vi "stopSel.vi"(5 "Der Ampl":dbl, 6 "Tipo":enum16{"Amplitud", "Fase", "Mixto"}(ring), 7 "Der Fase":dbl, 8 "thr":dbl, 9 "thr. Ang":dbl, 10 "Err.Amp":dbl, 11 "DifFase":dbl) -> (2 "stop":bool)   [LabVIEW 2018]
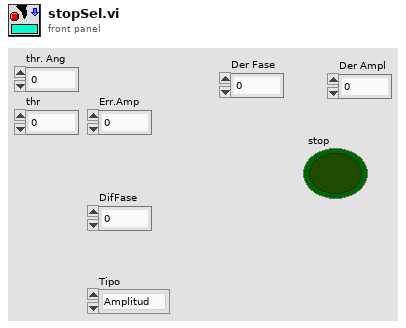
[diagram p1: front panel]
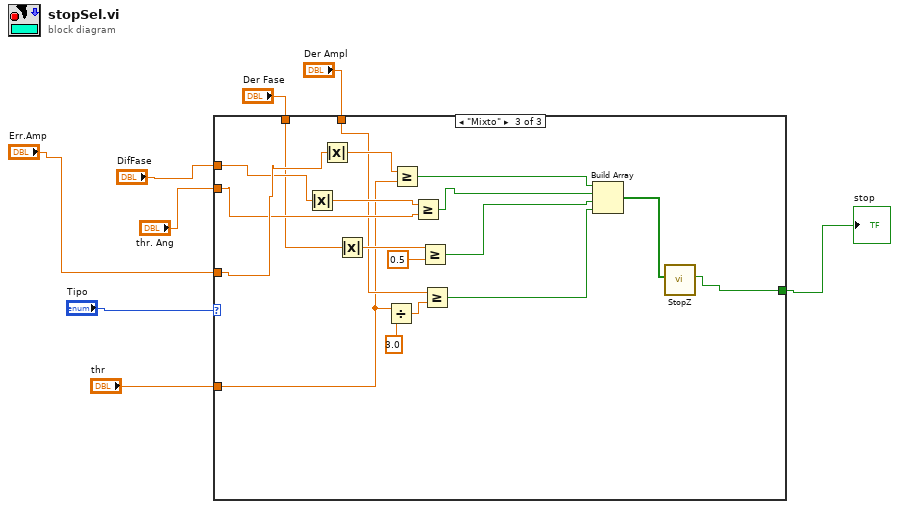
[diagram p0: block diagram]
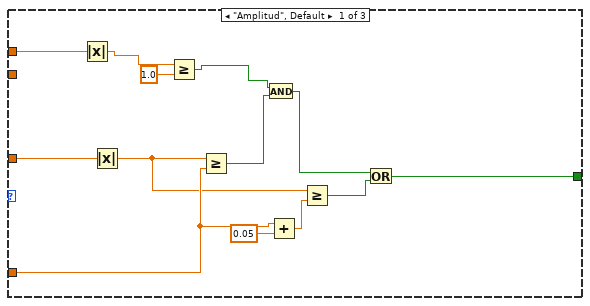
[diagram p2: hidden frame]
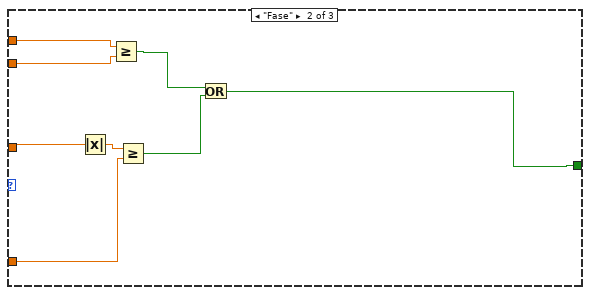
[diagram p3: hidden frame]
diagram:
  n1 = case shown="\"Mixto\"" "Tipo" {
    tunnel: "DifFase" -> [w21 w29 w42]
    tunnel: "thr. Ang" -> [_ w28 w40]
    tunnel: "Err.Amp" -> [w10 w26 w44]
    tunnel: "thr" -> [w14 w25 w32]
    tunnel: [w12 w22 w47] -> w3
    tunnel: "Der Fase" -> [_ _ w38]
    tunnel: "Der Ampl" -> [_ _ w34]
    frame "Amplitud", Default {
      n2 = Absolute Value(x=w21) -> (abs(x)=w20:dbl)
      n3 = Absolute Value(x=w10) -> (abs(x)=w9:dbl)
      n4 = Greater Or Equal?(x=w20, y=1.0) -> (x >= y?=w19:bool)
      n5 = Greater Or Equal?(x=w9, y=w14) -> (x >= y?=w18:bool)
      n6 = And(x=w19, y=w18) -> (x .and. y?=w17:bool)
      n7 = Add(x=w14, y=0.05) -> (x+y=w15:dbl)
      n8 = Greater Or Equal?(x=w9, y=w15) -> (x >= y?=w16:bool)
      n9 = Or(x=w17, y=w16) -> (x .or. y?=w12:bool)
    }
    frame "Fase" {
      n10 = Absolute Value(x=w26) -> (abs(x)=w27:dbl)
      n11 = Greater Or Equal?(x=w29, y=w28) -> (x >= y?=w24:bool)
      n12 = Greater Or Equal?(x=w27, y=w25) -> (x >= y?=w23:bool)
      n13 = Or(x=w24, y=w23) -> (x .or. y?=w22:bool)
    }
    frame "Mixto" {
      n14 = Absolute Value(x=w42) -> (abs(x)=w41:dbl)
      n15 = Absolute Value(x=w44) -> (abs(x)=w43:dbl)
      n16 = Absolute Value(x=w38) -> (abs(x)=w37:dbl)
      n17 = Divide(x=w32, y=3.0) -> (x/y=w33:dbl)
      n18 = Greater Or Equal?(x=w43, y=w32) -> (x >= y?=w46:bool)
      n19 = Greater Or Equal?(x=w41, y=w40) -> (x >= y?=w39:bool)
      n20 = Greater Or Equal?(x=w37, y=0.5) -> (x >= y?=w35:bool)
      n21 = Greater Or Equal?(x=w34, y=w33) -> (x >= y?=w30:bool)
      n22 = Build Array(w46, w39, w35, w30) -> (w45:bool[])
      n23 = call "StopZ.vi"("Optciones"=w45) -> ("parar"=w47:bool)  [unwired: 10 in]
    }
  }
  "stop" <- w3
